vi "main_cn.vi"() -> ()   [LabVIEW 2016]
uses:
  Controls/ExtRefSource.ctl
  Controls/Auto range.ctl
  UI functions/Main_UI_Var.ctl
  <instrlib>/Zurich Instruments LabOne/Public/ziTypeHandle.ctl
  Controls/zi_node.ctl
  UI functions/Main_FUN-Numeric_Var.ctl
  <instrlib>/Zurich Instruments LabOne/Public/Data/ziTypeDemodSampleSingle.ctl
  <instrlib>/Zurich Instruments LabOne/Public/Configure/ziSetValueDouble.vi
  <instrlib>/Zurich Instruments LabOne/Public/Configure/ziSetValueDoubleArray.vi
  <instrlib>/Zurich Instruments LabOne/Zurich Instruments LabOne.lvlib
panel:
  out "Label.Text":string
  in  "FUN-Numeric_Var":T1 {"ZI Handle"."Handle" format="0x%08x"; "ZI Handle"."Conn" format="0x%08x"}
  in  "sigouts/0/imp50":bool caption="50 Ω"
  in  "Address":string="DEV3505"
  in  "stop":bool
  in  "extrefs/0/enable":T4 caption="参考时钟"
  in  "Offset":dbl format="%#_3p"
  in  "Enable":bool
  in  "sigins/0/float":bool caption="Float"
  in  "sigins/0/diff":bool caption="差分"
  in  "sigins/0/imp50":bool caption="50 Ω"
  in  "sigins/0/ac":bool caption="AC"
  in  "sigins/0/autorange":T5=TRUE caption="Boolean"
  in  "sigouts/0/amplitudes/0":dbl=1.0 caption="输出幅值" format="%.2p Vpk"
  in  "sigouts/0/offset":dbl caption="偏置" format="%.2p V"
  in  "sigouts/0/range":dbl(ring)=1.0 caption="输出范围" items=["10 mV"=0.01, "100 mV"=0.1, "1 V"=1.0, "10 V"=10.0]
  in  "sigouts/0/enables/0":bool caption="启用"
  in  "demods/0/rate":dbl=52.31584930419922 caption="数据传输速率" format="%#.3p Sa/s"
  in  "sigouts/0/on":bool caption="启用"
  out "Title_SIG OUT":string
  out "Title_Demodulators":string
  out "Top_Left":bool
  in  "oscs/0/freq":dbl=99999.99999990905 caption="频率" format="%.8p"
  in  "demods/0/timeconstant":dbl(slide)=0.001 caption="时间常数" scale=3e-07..2.0
  in  "demods/0/harmonic":dbl=1.0 caption="谐波" min=1.0 max=1000.0 step=1.0 format="%#_1g"
  in  "demods/0/order":dbl(ring)=4.0 caption="阶次" items=["1"=1.0, "2"=2.0, "3"=3.0, "4"=4.0, "5"=5.0, "6"=6.0, "7"=7.0, "8"=8.0]
  in  "sigins/0/range":dbl=1.0 caption="量程" format="%.1p V"
  in  "参考时钟":u16(ring) items=["Internal Ref", "External Ref/Aux", "External Ref/DIO", "External Ref/Trigger"]
  out "Title_SIG IN":string
  out "Mid_Left":bool
  in  "UI_Var":T6 caption="Var" {"ZI Handle"."Handle" format="0x%08x"; "ZI Handle"."Conn" format="0x%08x"}
  out "X":dbl format="%.5p V"
  out "Mid_Mid":bool caption="Mid_Left"
  out "Y":dbl format="%.5p V"
  out "Mid_Right":bool caption="Mid_Left"
  in  "Preset":u16(ring) items=["Cartesian", "Polar"]
  out "Scope 3":dbl[](graph)
  out "Bottom_Left":bool caption="Mid_Left"
  out "Plotter(R&theta)":waveform(dbl)[](graph) caption="Plotter"
  out "Bottom_Right":bool caption="Mid_Left"
  out "Plotter(XY)":waveform(dbl)[](graph) caption="Plotter"
  # "For development only"
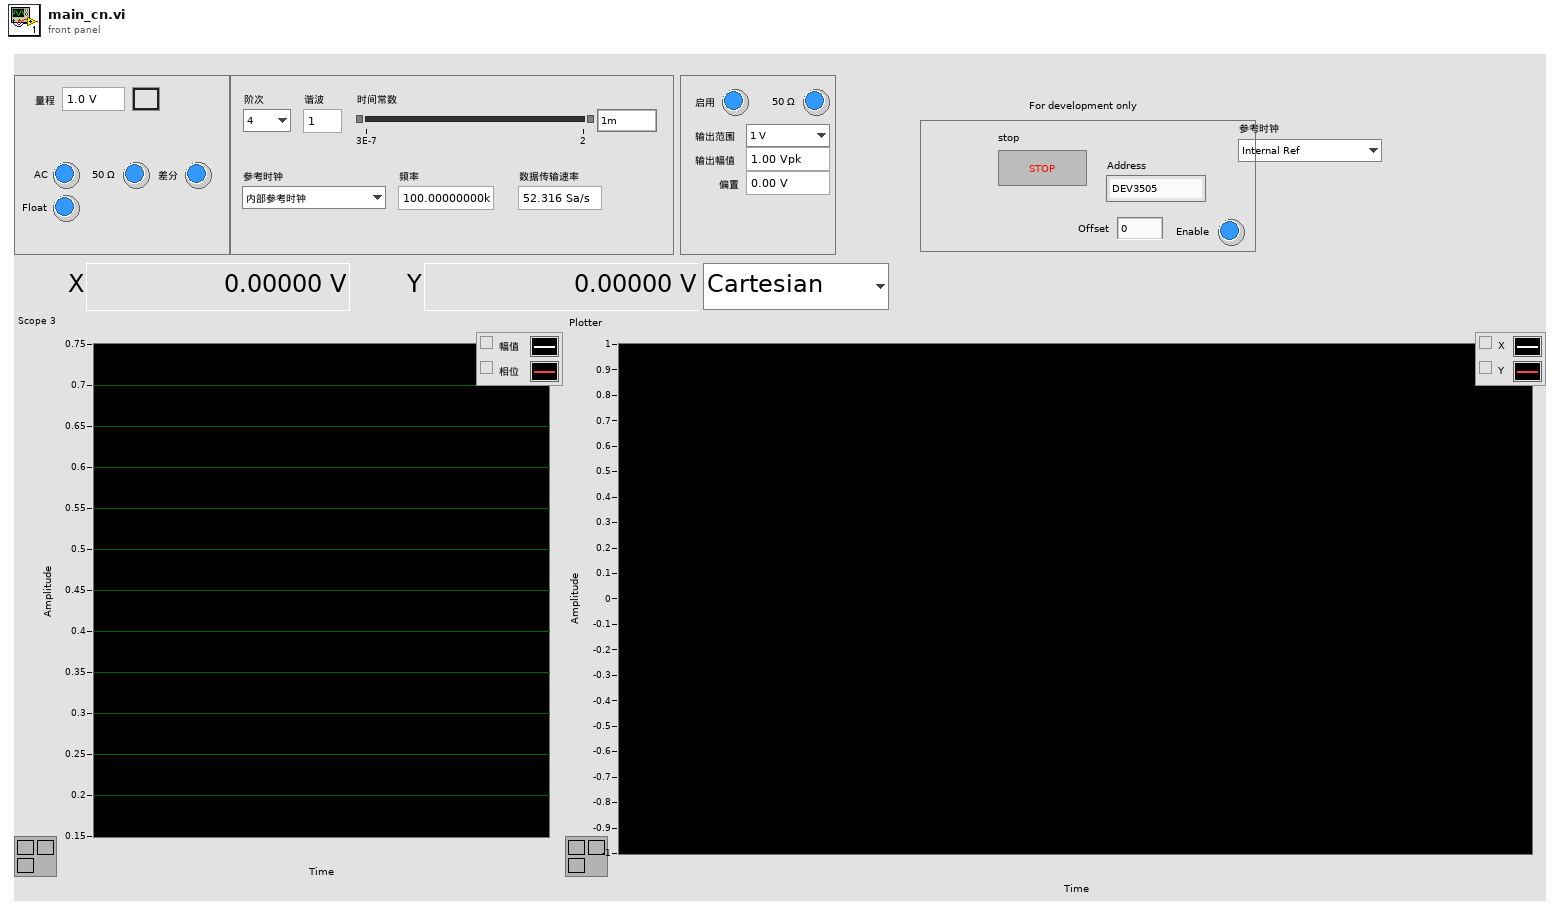
[diagram p1: front panel]
types:
  T1 = typedef "Main_FUN-Numeric_Var.ctl" = cluster{"ZI Handle":T2, "Demod Sample":T3}
  T2 = typedef "Zurich Instruments LabOne.lvlib/ziTypeHandle.ctl" = cluster{"handleValid":bool, "Conn":u64, "Path Prefix":string, "Handle":u64, "Connected":bool, "Clockbase(s)":dbl}
  T3 = typedef "Zurich Instruments LabOne.lvlib/ziTypeDemodSampleSingle.ctl" = cluster{"Timestamps (ticks)":u64, "X (Vrms)":dbl, "Y (Vrms)":dbl, "Osc Phase (deg)":dbl, "Freq (Hz)":dbl, "DIO":u32, "AuxIn0 (V)":dbl, "AuxIn1 (V)":dbl, "Trigger":u32}
  T4 = typedef "ExtRefSource.ctl" = enum16{"内部参考时钟", "外部参考时钟/Aux Input 1", "外部参考时钟/Trigger 1"}
  T5 = typedef "Auto range.ctl" = bool
  T6 = typedef "Main_UI_Var.ctl" = cluster{"ZI Handle":T2, "ZI_node":T7}
  T7 = typedef "zi_node.ctl" = cluster{"Node":string[], "Value":dbl[]}
  T8 = typedef "UI_Queue_Data Type" = cluster{"Cmd":string, "Value":variant}
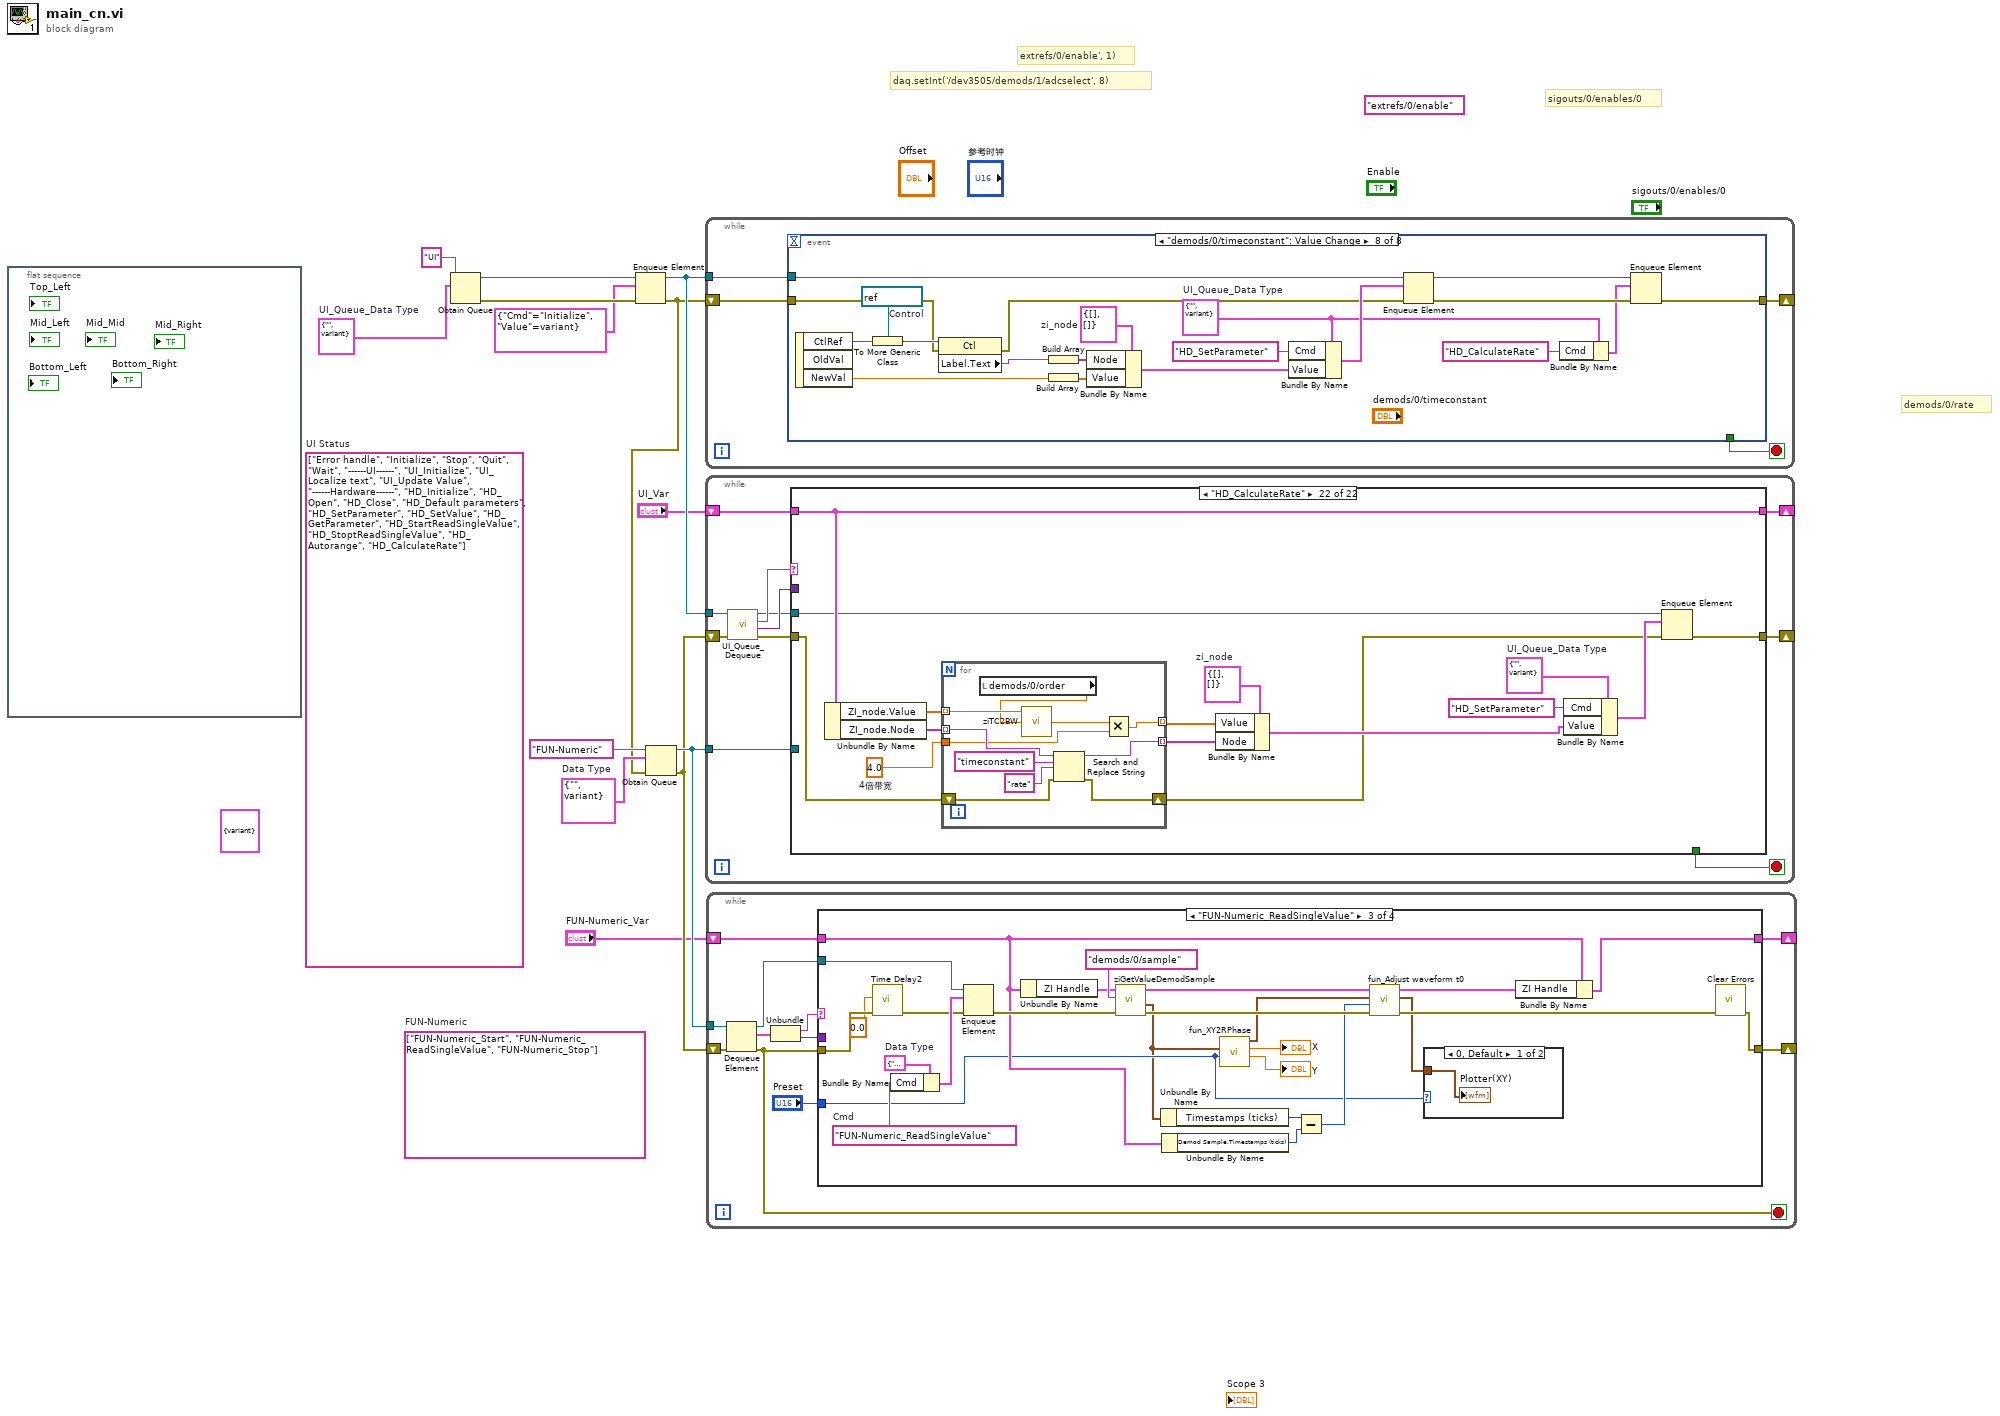
[diagram p0: block diagram]
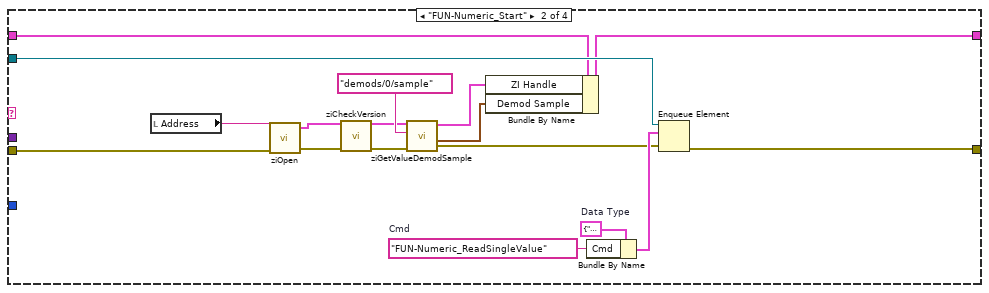
[diagram p3: hidden frame]
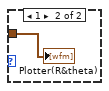
[diagram p4: hidden frame]
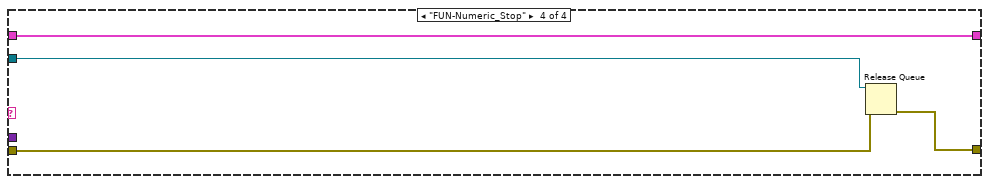
[diagram p5: hidden frame]
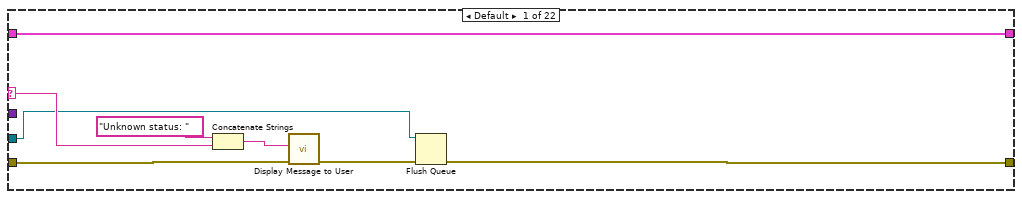
[diagram p6: hidden frame]
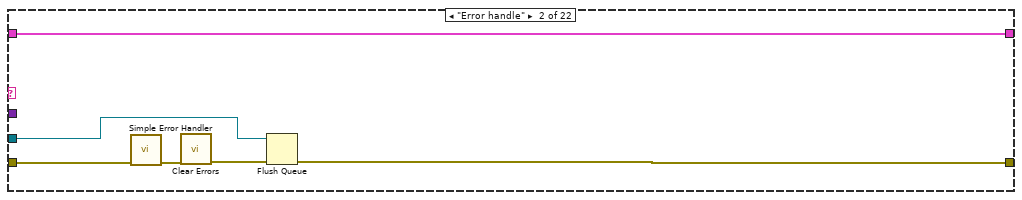
[diagram p7: hidden frame]
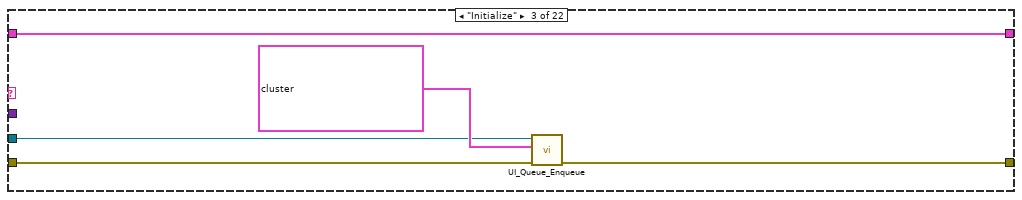
[diagram p8: hidden frame]
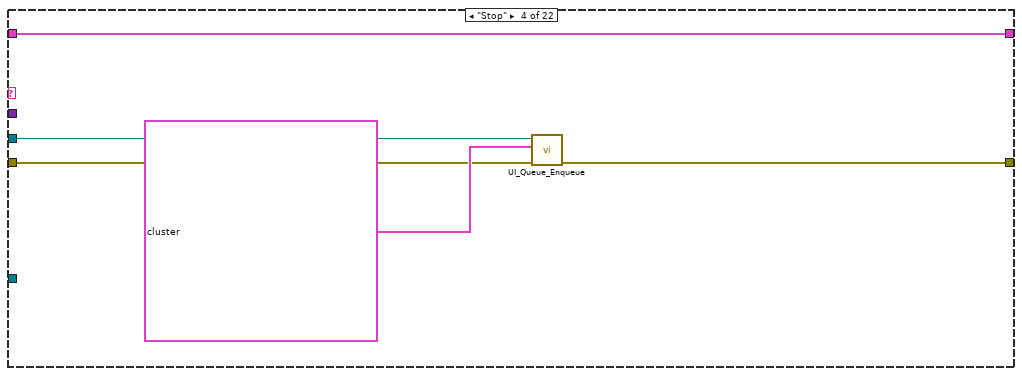
[diagram p9: hidden frame]
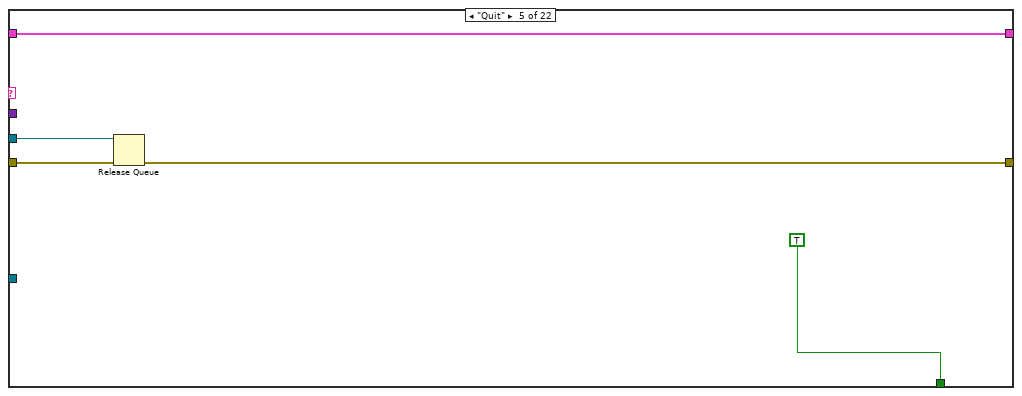
[diagram p10: hidden frame]
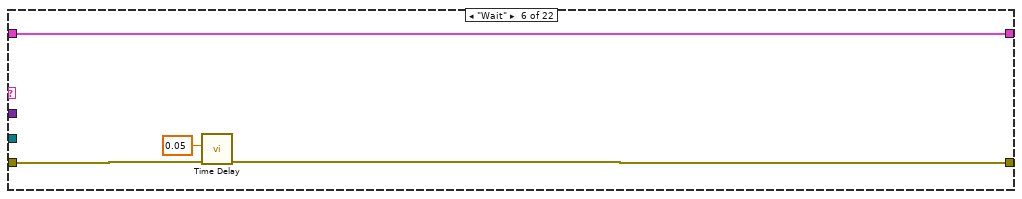
[diagram p11: hidden frame]
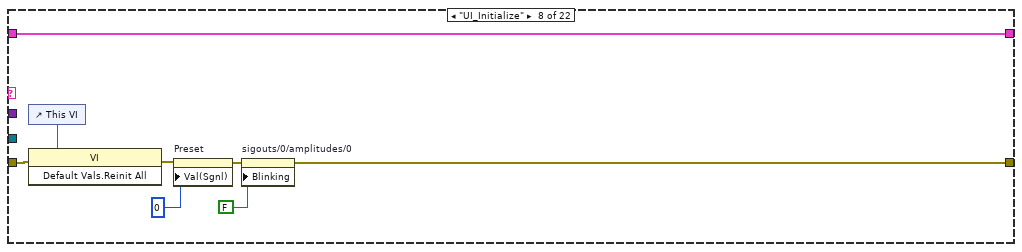
[diagram p13: hidden frame]
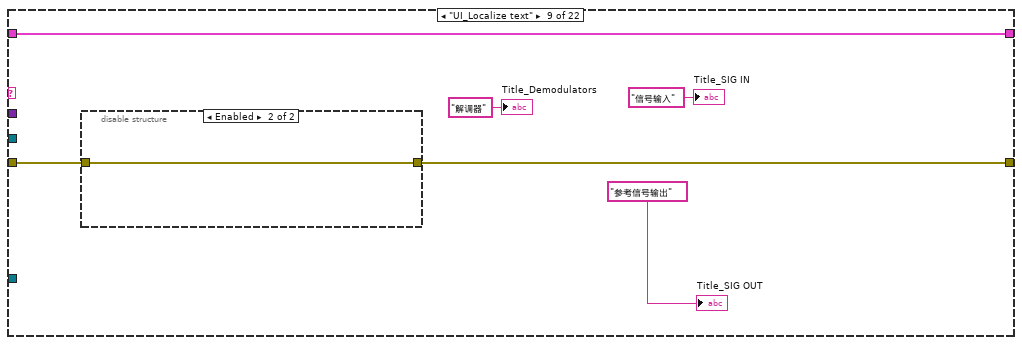
[diagram p14: hidden frame]
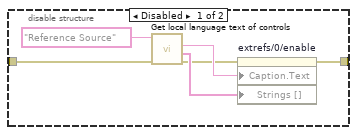
[diagram p15: hidden frame]
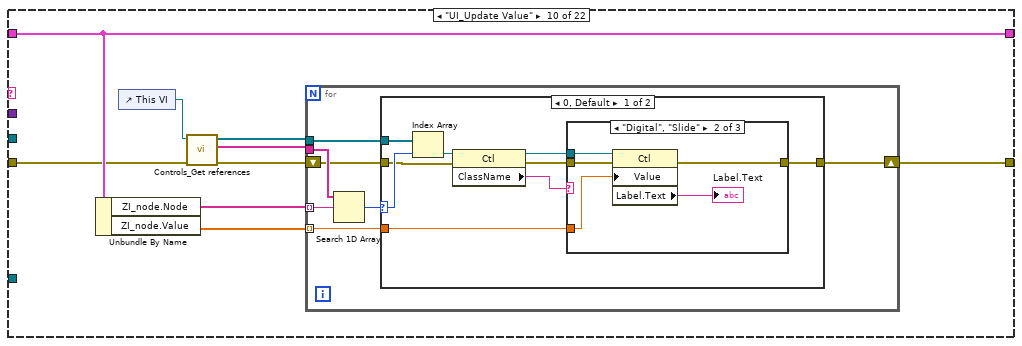
[diagram p16: hidden frame]
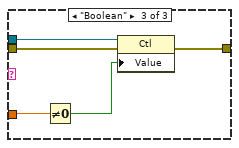
[diagram p18: hidden frame]
diagram:
  (unwired) "extrefs/0/enable"
  w5 = cluster{"Cmd":string, "Value":variant} {"Cmd"="", "Value"=variant}  # Data Type
  (unwired) cluster{"Value":variant} {"Value"=variant} ("element")
  (unwired) string[] ["FUN-Numeric_Start", "FUN-Numeric_ReadSingleValue", "FUN-Numeric_Stop"]  # FUN-Numeric
  (unwired) string[] ["Error handle", "Initialize", "Stop", "Quit", "Wait", "------UI------", "UI_Initialize", "UI_Localize text", "UI_Update Value", "------Hardware------", "HD_Initialize", "HD_Open", "HD_Close", "HD_Default parameters", "HD_SetParameter", "HD_SetValue", "HD_GetParameter", "HD_StartReadSingleValue", "HD_StoptReadSingleValue", "HD_Autorange", "HD_CalculateRate"]  # UI Status
  w6 = T8 {"Cmd"="", "Value"=variant}  # UI_Queue_Data Type
  # "daq.setInt('/dev3505/demods/1/adcselect', 8)"
  # "extrefs/0/enable', 1)"
  # "demods/0/rate"
  # "sigouts/0/enables/0"
  n1 = flat-sequence {
    frame #0 {
    }
  }
  n2 = Obtain Queue(name (unnamed)="UI", element data type=w6) -> (queue out=w12:refnum<queue>, error out=w11:errorcluster)  [unwired: 3 in, 1 out]
  n3 = Enqueue Element(queue=w12, element=cluster{"Cmd":string, "Value":variant} {"Cmd"="Initialize", "Value"=variant}, error in (no error)=w11) -> (queue out=w10:refnum<queue>, error out=w2:errorcluster)  [unwired: 1 in, 1 out]
  n4 = Obtain Queue(name (unnamed)="FUN-Numeric", element data type=w5, error in (no error)=w2) -> (queue out=w4:refnum<queue>, error out=w3:errorcluster)  [unwired: 2 in, 1 out]
  n5 = while {
    tunnel: w10 -> [w17]
    shift-right: [w14] -> _
    shift-left: w2 -> [w15]
    stop <- w16 stop-if-true
    n6 = event shown="[7] \"demods/0/timeconstant\": Value Change" {
      selector: _ -> [_ _ _ _ _ _ _ _]
      dyn-events: _ -> [_ _ _ _ _ _ _ _]
      timeout: _ -> [_ _ _ _ _ _ _ _]
      tunnel: [_ "stop" _ _ _ _ _ _] -> w16
      tunnel: w17 -> [_ w22 _ w59 w76 w91 w102 w122]
      tunnel: w15 -> [w18 w20 _ w43 w64 w78 w95 w111]
      tunnel: [w18 w19 _ w49 w69 _ _ w104] -> w14
      event Timeout {
        n7 = event-data() -> ()  [unwired: 1 in, 3 out]
      }
      event "stop": Value Change {
        n8 = event-data() -> ()  [unwired: 1 in, 6 out]
        n9 = Enqueue Element(queue=w22, element=cluster{"Cmd":string, "Value":variant} {"Cmd"="Stop", "Value"=variant}, error in (no error)=w20) -> (error out=w19:errorcluster)  [unwired: 1 in, 2 out]
      }
      event "Preset": Value Change {
        n10 = event-data() -> ("NewVal"=w26:u16)  [unwired: 1 in]
        n11 = invoke on="Plotter(XY)" class="WFChart (strict)" method="Reinit To Default"() -> ()  [unwired: 3 in, 3 out]
        n12 = case shown="0, Default" w26 {
          tunnel: ["%.5p V" "%.5p V"] -> w30
          tunnel: ["%.5p deg" "%.5p V"] -> w29
          tunnel: ["幅值" "X"] -> w28
          tunnel: ["相位" "Y"] -> w27
          frame 1 {
          }
          frame 0, Default {
          }
        }
        n13 = property on="X" class="DigNum (strict)"("Caption.Text"=w28) -> ()  [unwired: 2 in, 2 out]
        n14 = property on="Y" class="DigNum (strict)"("Caption.Text"=w27) -> ()  [unwired: 2 in, 2 out]
        n15 = property on="X" class="DigNum (strict)"("FormatString"=w30) -> ()  [unwired: 2 in, 2 out]
        n16 = property on="Y" class="DigNum (strict)"("FormatString"=w29) -> ()  [unwired: 2 in, 2 out]
        n17 = case shown="1" w26 {
          tunnel: [TRUE FALSE] -> w25
          tunnel: [FALSE TRUE] -> w24
          frame 0, Default {
          }
          frame 1 {
          }
        }
        n18 = property on="Plotter(XY)" class="WFChart (strict)"("Visible"=w25) -> ()  [unwired: 2 in, 2 out]
        n19 = property on="Plotter(R&theta)" class="WFChart (strict)"("Visible"=w24) -> ()  [unwired: 2 in, 2 out]
      }
      event "sigouts/0/on", "sigins/0/diff", "sigins/0/imp50", "sigins/0/ac", "sigouts/0/imp50", "sigins/0/float": Value Change {
        w47 = refnum<vi> refnum  # Control
        w53 = T8 {"Cmd"="", "Value"=variant}  # UI_Queue_Data Type
        w58 = T7 {"Node"=[], "Value"=[]}  # zi_node
        n20 = event-data() -> ("CtlRef"=w46:refnum<vi>, "NewVal"=w56:bool)  [unwired: 1 in, 4 out]
        n21 = To More Generic Class(target class=w47, reference=w46) -> (generic class reference=w48:refnum<vi>)
        n22 = property class="Ctl"(reference=w48, error in=w43) -> (error out=w44:errorcluster, "Label.Text"=w45:string)  [unwired: 1 out]
        n23 = Boolean To (0,1)(Boolean=w56) -> (0, 1=w54:i16)
        n24 = Build Array(w45) -> (w57:string[])
        n25 = Build Array(w54) -> (w55:i16[])
        n26 = Bundle By Name(cluster=w58, "Node"=w57, "Value"=w55) -> (w51:T7)
        n27 = Bundle By Name(cluster=w53, "Cmd"="HD_SetParameter", "Value"=w51) -> (w52:T8)
        n28 = Enqueue Element(queue=w59, element=w52, error in (no error)=w44) -> (error out=w49:errorcluster)  [unwired: 1 in, 2 out]
      }
      event Value Change {
        w67 = refnum<vi> refnum  # Control
        w73 = T8 {"Cmd"="", "Value"=variant}  # UI_Queue_Data Type
        w75 = T7 {"Node"=[], "Value"=[]}  # zi_node
        # "sigins/0/autorange"
        n29 = event-data() -> ("CtlRef"=w66:refnum<vi>)  [unwired: 1 in, 3 out]
        n30 = To More Generic Class(target class=w67, reference=w66) -> (generic class reference=w68:refnum<vi>)
        n31 = property class="Ctl"(reference=w68, error in=w64) -> (error out=w65:errorcluster, "Label.Text"=w61:string)  [unwired: 1 out]
        n32 = Match Pattern(string=w61, regular expression="sigins/[0-9]") -> (match substring=w60:string)  [unwired: 1 in, 3 out]
        n33 = Build Array(w60) -> (w74:string[])
        n34 = Bundle By Name(cluster=w75, "Node"=w74, "Value"=dbl[] [1.0]) -> (w71:T7)
        n35 = Bundle By Name(cluster=w73, "Cmd"="HD_Autorange", "Value"=w71) -> (w72:T8)
        n36 = Enqueue Element(queue=w76, element=w72, error in (no error)=w65) -> (error out=w69:errorcluster)  [unwired: 1 in, 2 out]
      }
      event "sigouts/0/amplitudes/0", "demods/0/rate", "oscs/0/freq", "demods/0/order", "demods/0/harmonic", "sigins/0/range", "sigouts/0/range", "sigouts/0/offset": Value Change {
        w80 = refnum<vi> refnum  # Control
        w88 = T8 {"Cmd"="", "Value"=variant}  # UI_Queue_Data Type
        w90 = T7 {"Node"=[], "Value"=[]}  # zi_node
        n37 = event-data() -> ("CtlRef"=w82:refnum<vi>, "NewVal"=w84:dbl)  [unwired: 1 in, 4 out]
        n38 = To More Generic Class(target class=w80, reference=w82) -> (generic class reference=w81:refnum<vi>)
        n39 = property class="Ctl"(reference=w81, error in=w78) -> (error out=w77:errorcluster, "Label.Text"=w79:string)  [unwired: 1 out]
        n40 = Build Array(w79) -> (w89:string[])
        n41 = Build Array(w84) -> (w83:dbl[])
        n42 = Bundle By Name(cluster=w90, "Node"=w89, "Value"=w83) -> (w86:T7)
        n43 = Bundle By Name(cluster=w88, "Cmd"="HD_SetParameter", "Value"=w86) -> (w87:T8)
        n44 = Enqueue Element(queue=w91, element=w87, error in (no error)=w77) -> ()  [unwired: 1 in, 3 out]
      }
      event Value Change {
        w96 = refnum<vi> refnum  # Control
        w101 = T8 {"Cmd"="", "Value"=variant}  # UI_Queue_Data Type
        n45 = event-data() -> ("CtlRef"=w98:refnum<vi>, "NewVal"=w93:T4)  [unwired: 1 in, 4 out]
        n46 = To More Generic Class(target class=w96, reference=w98) -> (generic class reference=w97:refnum<vi>)
        n47 = property class="Ctl" props=["Label", "Text"](reference=w97, error in=w95) -> (error out=w94:errorcluster)  [unwired: 2 out]
        n48 = call "ExtRefSource_set.vi"("extrefs/0/enable"=w93) -> ("zi_node"=w92:T7)  [unwired: 10 in]
        n49 = Bundle By Name(cluster=w101, "Cmd"="HD_SetParameter", "Value"=w92) -> (w100:T8)
        n50 = Enqueue Element(queue=w102, element=w100, error in (no error)=w94) -> ()  [unwired: 1 in, 3 out]
      }
      event "demods/0/timeconstant": Value Change {
        w112 = refnum<vi> refnum  # Control
        w107 = T8 {"Cmd"="", "Value"=variant}  # UI_Queue_Data Type
        w121 = T7 {"Node"=[], "Value"=[]}  # zi_node
        n51 = event-data() -> ("CtlRef"=w114:refnum<vi>, "NewVal"=w116:dbl)  [unwired: 1 in, 1 out]
        n52 = To More Generic Class(target class=w112, reference=w114) -> (generic class reference=w113:refnum<vi>)
        n53 = property class="Ctl"(reference=w113, error in=w111) -> (error out=w110:errorcluster, "Label.Text"=w109:string)  [unwired: 1 out]
        n54 = Build Array(w109) -> (w120:string[])
        n55 = Build Array(w116) -> (w115:dbl[])
        n56 = Bundle By Name(cluster=w121, "Node"=w120, "Value"=w115) -> (w118:T7)
        n57 = Bundle By Name(cluster=w107, "Cmd"="HD_SetParameter", "Value"=w118) -> (w119:T8)
        n58 = Enqueue Element(queue=w122, element=w119, error in (no error)=w110) -> (queue out=w106:refnum<queue>, error out=w105:errorcluster)  [unwired: 1 in, 1 out]
        n59 = Bundle By Name(cluster=w107, "Cmd"="HD_CalculateRate") -> (w103:T8)
        n60 = Enqueue Element(queue=w106, element=w103, error in (no error)=w105) -> (error out=w104:errorcluster)  [unwired: 1 in, 2 out]
      }
    }
  }
  n61 = while {
    tunnel: w10 -> [w133]
    shift-right: [w127] -> _
    shift-left: w3 -> [w132]
    shift-right: [w124] -> _
    shift-left: "UI_Var" -> [w125]
    tunnel: w4 -> [w123]
    stop <- w126 stop-if-true
    n62 = call "UI_Queue_Dequeue.vi"("error in (no error)"=w132, "UI Queue in"=w133) -> ("error out"=w130:errorcluster, "Value"=w129:variant, "Cmd"=w131:string, "UI Queue out"=w128:refnum<queue>)  [unwired: 6 in]
    n63 = case shown="\"HD_CalculateRate\"" w131 {
      selector: w131 -> [w140 _ _ _ _ _ _ _ _ _ _ _ _ _ _ _ _ _ _ _ _ _]
      tunnel: w130 -> [w141 w147 w151 w156 w162 w165 w168 w172 w179 w190 w228 w232 w240 w246 w257 w270 w286 w299 w308 w316 w336 w349]
      tunnel: w129 -> [_ _ _ _ _ _ _ _ _ _ _ _ _ _ _ _ w293 _ _ _ w335 _]
      tunnel: w128 -> [w138 w143 w149 w154 w161 _ _ _ _ _ _ w229 _ _ w250 w272 w288 _ _ _ w325 w356]
      tunnel: [w139 w144 w150 w155 w160 w164 w168 w170 w178 w192 w228 w231 w236 w245 w252 w273 w290 w300 w311 w315 w323 w355] -> w127
      tunnel: [_ _ _ _ TRUE _ _ _ _ _ _ _ _ _ _ _ _ _ _ _ _ _] -> w126
      tunnel: w125 -> [w137 w142 w148 w153 w158 w166 w167 w176 w177 w191 w227 w233 w239 w243 w260 w271 w289 w306 w312 w320 w334 w359]
      tunnel: [w137 w142 w148 w153 w158 w166 w167 w176 w177 w191 w227 w233 w238 w247 w261 w269 w285 w304 w312 w320 w330 w359] -> w124
      tunnel: w123 -> [_ _ _ _ _ _ _ _ _ _ _ _ _ _ _ _ _ _ w309 w314 _ _]
      frame Default {
        n64 = Concatenate Strings("Unknown status: " ("string"), w140) -> (w136:string)
        n65 = call "Display Message to User"("error in (no error)"=w141, "Message"=w136) -> ("error out"=w134:errorcluster)  [unwired: 8 in, 1 out]
        n66 = Flush Queue(queue=w138, error in (no error)=w134) -> (error out=w139:errorcluster)  [unwired: 2 out]
      }
      frame "Error handle" {
        n67 = call <vilib>:"Simple Error Handler.vi"("error in (no error)"=w147) -> ("error out"=w146:errorcluster)  [unwired: 4 in, 4 out]
        n68 = call <vilib>:"Clear Errors.vi"("error in (no error)"=w146) -> ("error out"=w145:errorcluster)  [unwired: 5 in, 1 out]
        n69 = Flush Queue(queue=w143, error in (no error)=w145) -> (error out=w144:errorcluster)  [unwired: 2 out]
      }
      frame "Initialize" {
        n70 = call "UI_Queue_Enqueue.vi"("error in (no error)"=w151, "UI Commands"=cluster{"Cmd":string, "Value":variant}[] [{"Cmd"="UI_Initialize", "Value"=variant}, {"Cmd"="UI_Localize text", "Value"=variant}, {"Cmd"="HD_Initialize", "Value"=variant}], "Queue in"=w149) -> ("error out"=w150:errorcluster)  [unwired: 7 in, 1 out]
      }
      frame "Stop" {
        n71 = call "UI_Queue_Enqueue.vi"("error in (no error)"=w156, "UI Commands"=cluster{"Cmd":string, "Value":variant}[] [{"Cmd"="HD_StoptReadSingleValue", "Value"=variant}, {"Cmd"="HD_Close", "Value"=variant}, {"Cmd"="Quit", "Value"=variant}], "Queue in"=w154) -> ("error out"=w155:errorcluster)  [unwired: 7 in, 1 out]
      }
      frame "Quit" {
        n72 = Release Queue(queue=w161, error in (no error)=w162) -> (error out=w160:errorcluster)  [unwired: 1 in, 2 out]
      }
      frame "Wait" {
        n73 = call "Time Delay"("error in (no error)"=w165, "Delay Time (s)"=0.05) -> ("error out"=w164:errorcluster)  [unwired: 9 in]
      }
      frame "------UI------" {
      }
      frame "UI_Initialize" {
        n74 = control-ref of="This VI"() -> (w174:refnum<vi>)
        n75 = invoke class="VI" method="Default Vals.Reinit All"(reference=w174, error in=w172) -> (error out=w173:errorcluster)  [unwired: 1 in, 2 out]
        n76 = property on="Preset" class="Ring (strict)"(error in=w173, "Val(Sgnl)"=u16 0 ("Value (Signaling)")) -> (error out=w171:errorcluster)  [unwired: 1 in, 1 out]
        n77 = property on="sigouts/0/amplitudes/0" class="DigNum (strict)"(error in=w171, "Blinking"=FALSE) -> (error out=w170:errorcluster)  [unwired: 1 in, 1 out]
      }
      frame "UI_Localize text" {
        n78 = disable-structure shown="Enabled" {
          disable-tunnel: w179 -> [w184 w189]
          disable-tunnel: [w183 w189] -> w178
          frame Disabled {
            n79 = call "Get local language text of controls.vi"("error in (no error)"=w184, "Control Label"="Reference Source") -> ("error out"=w185:errorcluster, "Values"=w187:string[], "Control Caption"=w186:string)  [unwired: 6 in, 1 out]
            n80 = property on="extrefs/0/enable" class="Enum (strict)"(error in=w185, "Caption.Text"=w186, "Strings []"=w187) -> (error out=w183:errorcluster)  [unwired: 1 in, 1 out]
          }
          frame Enabled {
          }
        }
        "Title_SIG IN" <- "信号输入" ("Title_SIG IN")
        "Title_Demodulators" <- "解调器" ("Title_SIG IN 2")
        "Title_SIG OUT" <- "参考信号输出" ("Title_SIG OUT")
      }
      frame "UI_Update Value" {
        n81 = Unbundle By Name(w191) -> ("ZI_node.Node"=w197:string[], "ZI_node.Value"=w193:dbl[])
        n82 = control-ref of="This VI"() -> (w198:refnum<vi>)
        n83 = call "Controls_Get references.vi"("error in (no error)"=w190, "VI in"=w198) -> ("error out"=w194:errorcluster, "Labels of Controls"=w196:string[], "References of Controls"=w195:refnum<vi>[])  [unwired: 7 in]
        n84 = for {
          tunnel: w197 -> [w204] mode=indexing
          tunnel: w196 -> [w205]
          tunnel: w195 -> [w202]
          tunnel: w193 -> [w200] mode=indexing
          shift-right: [w199] -> w192
          shift-left: w194 -> [w201]
          n85 = Search 1D Array(1D array=w205, element=w204) -> (index of element=w203:i32)  [unwired: 1 in]
          n86 = case shown="0, Default" w203 {
            selector: w203 -> [w214 _]
            tunnel: w202 -> [w213 _]
            tunnel: w201 -> [w212 w226]
            tunnel: w200 -> [w206 _]
            tunnel: [w209 w226] -> w199
            frame 0, Default {
              n87 = Index Array(array=w213, index=w214) -> (element=w211:refnum<vi>)
              n88 = property class="Ctl"(reference=w211, error in=w212) -> (reference out=w208:refnum<vi>, error out=w210:errorcluster, "ClassName"=w207:string)
              n89 = case shown="\"Digital\", \"Slide\"" w207 {
                tunnel: w210 -> [w215 w220 w225]
                tunnel: [w215 w219 w224] -> w209
                tunnel: w208 -> [_ w218 w223]
                tunnel: w206 -> [_ w217 w222]
                frame Default {
                }
                frame "Digital", "Slide" {
                  n90 = property class="Ctl"(reference=w218, error in=w220, "Value"=w217) -> (error out=w219:errorcluster, "Label.Text"=→"Label.Text":string)  [unwired: 1 out]
                }
                frame "Boolean" {
                  n91 = Not Equal To 0?(x=w222) -> (x != 0?=w221:bool)
                  n92 = property class="Ctl"(reference=w223, error in=w225, "Value"=w221) -> (error out=w224:errorcluster)  [unwired: 1 out]
                }
              }
            }
            frame -1 {
            }
          }
        }
      }
      frame "------Hardware------" {
      }
      frame "HD_Initialize" {
        # "HD_StartReadSingleValue"
        n93 = call "UI_Queue_Enqueue.vi"("error in (no error)"=w232, "UI Commands"=cluster{"Cmd":string, "Value":variant}[] [{"Cmd"="HD_Open", "Value"=variant}, {"Cmd"="HD_Default parameters", "Value"=variant}, {"Cmd"="HD_StartReadSingleValue", "Value"=variant}], "Queue in"=w229) -> ("error out"=w231:errorcluster)  [unwired: 7 in, 1 out]
      }
      frame "HD_Open" {
        n94 = call <instrlib>:"ziOpen.vi"("Error In"=w240, "Address"="Address") -> ("Error Out"=w237:errorcluster, "HandleOut"=w235:T2)  [unwired: 2 in, 1 out]
        n95 = call <instrlib>:"ziCheckVersion.vi"("Handle In"=w235, "Error In"=w237) -> ("Handle Out"=w234:T2, "Error Out"=w236:errorcluster)  [unwired: 11 in, 1 out]
        n96 = Bundle By Name(cluster=w239, "ZI Handle"=w234) -> (w238:T6)
      }
      frame "HD_Close" {
        n97 = Unbundle By Name(w243) -> ("ZI Handle"=w242:T2)
        n98 = call <instrlib>:"ziClose.vi"("Error In"=w246, "Handle In"=w242) -> ("Error Out"=w245:errorcluster, "Handle Out"=w244:T2)  [unwired: 2 in]
        n99 = Bundle By Name(cluster=w243, "ZI Handle"=w244) -> (w247:T6)
      }
      frame "HD_Default parameters" {
        n100 = Unbundle By Name(w260) -> ("ZI Handle"=w258:T2)
        n101 = call-poly <instrlib>:"ziSetValue.vi"("Error In"=w257, "Value"=0.0, "Path"="sigouts/0/on", "Handle In"=w258) -> ("Error Out"=w256:errorcluster, "Handle Out"=w248:T2)  [unwired: 1 in]
        n102 = call "Lock-in Default parameters.vi"("error in (no error)"=w256, "Handle in"=w248) -> ("error out"=w251:errorcluster, "zi_node"=w249:T7, "Handle out"=w259:T2)  [unwired: 7 in]
        n103 = Bundle By Name(cluster=w260, "ZI Handle"=w259, "ZI_node"=w249) -> (w261:T6)
        n104 = for {
          tunnel: cluster{"Cmd":string, "Value":variant}[] [{"Cmd"="HD_GetParameter", "Value"=variant}, {"Cmd"="Wait", "Value"=variant}] ("UI Commands") -> [w265] mode=indexing
          tunnel: w250 -> [w262]
          shift-right: [w264] -> w252
          shift-left: w251 -> [w263]
          n105 = Enqueue Element At Opposite End(queue=w262, element=w265, error in (no error)=w263) -> (error out=w264:errorcluster)  [unwired: 1 in, 2 out]
        }
      }
      frame "HD_GetParameter" {
        n106 = Unbundle By Name(w271) -> ("ZI_node.Node"=w267:string[])
        n107 = for {
          tunnel: w267 -> [w280] mode=indexing
          shift-right: [w282] -> w274
          shift-left: w270 -> [w283]
          tunnel: [w279] -> w266 mode=indexing
          shift-right: [w277] -> w275
          shift-left: w271 -> [w278]
          n108 = Unbundle By Name(w278) -> ("ZI Handle"=w281:T2)
          n109 = call <instrlib>:"ziGetValueDouble.vi"("error in"=w283, "Path"=w280, "Handle in"=w281) -> ("error out"=w282:errorcluster, "Value"=w279:dbl, "Handle out"=w276:T2)
          n110 = Bundle By Name(cluster=w278, "ZI Handle"=w276) -> (w277:T6)
        }
        n111 = Bundle By Name(cluster=w275, "ZI_node.Node"=w267, "ZI_node.Value"=w266) -> (w269:T6)
        n112 = Enqueue Element(queue=w272, element=cluster{"Cmd":string, "Value":variant} {"Cmd"="UI_Update Value", "Value"=variant}, error in (no error)=w274) -> (error out=w273:errorcluster)  [unwired: 1 in, 2 out]
      }
      frame "HD_SetParameter" {
        w292 = T7 {"Node"=[], "Value"=[]}  # zi_node
        n113 = Variant To Data(error in=w286, type=w292, Variant=w293) -> (data=w284:T7, error out=w287:errorcluster)
        n114 = Bundle By Name(cluster=w289, "ZI_node"=w284) -> (w285:T6)
        n115 = for {
          tunnel: cluster{"Cmd":string, "Value":variant}[] [{"Cmd"="HD_SetValue", "Value"=variant}, {"Cmd"="Wait", "Value"=variant}, {"Cmd"="HD_GetParameter", "Value"=variant}] ("UI Commands") -> [w295] mode=indexing
          shift-right: [w297] -> w290
          shift-left: w287 -> [w296]
          tunnel: w288 -> [w294]
          n116 = Enqueue Element(queue=w294, element=w295, error in (no error)=w296) -> (error out=w297:errorcluster)  [unwired: 1 in, 2 out]
        }
      }
      frame "HD_SetValue" {
        # "Can be replaced by \"Double Array\""
        n117 = Unbundle By Name(w306) -> ("ZI Handle"=w305:T2, "ZI_node"=w298:T7)
        n118 = Unbundle By Name(w298) -> ("Node"=w302:string[], "Value"=w303:dbl[])
        n119 = call-poly <instrlib>:"ziSetValue.vi"("Error In"=w299, "Values"=w303, "Paths"=w302, "Handle In"=w305) -> ("Error Out"=w300:errorcluster, "Handle Out"=w301:T2)  [unwired: 1 in]
        n120 = Bundle By Name(cluster=w306, "ZI Handle"=w301, "ZI_node"=w298) -> (w304:T6)
      }
      frame "HD_StartReadSingleValue" {
        w310 = cluster{"Cmd":string, "Value":variant} {"Cmd"="", "Value"=variant}  # Data Type
        w313 = "FUN-Numeric_Start"  # Cmd
        n121 = Bundle By Name(cluster=w310, "Cmd"=w313) -> (w307:cluster{"Cmd":string, "Value":variant})
        n122 = Enqueue Element(queue=w309, element=w307, error in (no error)=w308) -> (error out=w311:errorcluster)  [unwired: 1 in, 2 out]
      }
      frame "HD_StoptReadSingleValue" {
        w318 = cluster{"Cmd":string, "Value":variant} {"Cmd"="", "Value"=variant}  # Data Type
        w317 = "FUN-Numeric_Stop"  # Cmd
        n123 = Bundle By Name(cluster=w318, "Cmd"=w317) -> (w319:cluster{"Cmd":string, "Value":variant})
        n124 = Enqueue Element(queue=w314, element=w319, error in (no error)=w316) -> (error out=w315:errorcluster)  [unwired: 1 in, 2 out]
      }
      frame "HD_Autorange" {
        w327 = string[] ["sigins/0/range"]  # Read changed range
        w337 = T7 {"Node"=[], "Value"=[]}  # zi_node
        n125 = Variant To Data(error in=w336, type=w337, Variant=w335) -> (data=w333:T7, error out=w332:errorcluster)
        n126 = Unbundle By Name(w333) -> ("Node"=w328:string[])
        n127 = Unbundle By Name(w334) -> ("ZI Handle"=w331:T2)
        n128 = for {
          shift-right: [w345] -> w324
          shift-left: w332 -> [w346]
          shift-right: [w343] -> w329
          shift-left: w331 -> [w344]
          tunnel: w328 -> [w342] mode=indexing
          n129 = call <instrlib>:"ziAutoRange.vi"("Error in"=w346, "Path"=w342, "Handle in"=w344) -> ("Error out"=w345:errorcluster, "Handle out"=w343:T2)  [unwired: 6 in, 1 out]
        }
        n130 = call "Time Delay3"("error in (no error)"=w324, "Delay Time (s)"=0.5) -> ("error out"=w322:errorcluster)  [unwired: 9 in]
        n131 = Bundle By Name(cluster=w334, "ZI_node.Node"=w327, "ZI Handle"=w329) -> (w330:T6)
        n132 = for {
          tunnel: cluster{"Cmd":string, "Value":variant}[] [{"Cmd"="HD_GetParameter", "Value"=variant}, {"Cmd"="Wait", "Value"=variant}] ("UI Commands") -> [w339] mode=indexing
          shift-right: [w341] -> w323
          shift-left: w322 -> [w340]
          tunnel: w325 -> [w338]
          n133 = Enqueue Element(queue=w338, element=w339, error in (no error)=w340) -> (error out=w341:errorcluster)  [unwired: 1 in, 2 out]
        }
      }
      frame "HD_CalculateRate" {
        w347 = 4.0  # 4倍带宽
        w353 = T8 {"Cmd"="", "Value"=variant}  # UI_Queue_Data Type
        w354 = T7 {"Node"=[], "Value"=[]}  # zi_node
        n134 = Unbundle By Name(w359) -> ("ZI_node.Value"=w360:dbl[], "ZI_node.Node"=w361:string[])
        n135 = for {
          tunnel: w361 -> [w370] mode=indexing
          shift-right: [w368] -> w348
          shift-left: w349 -> [w369]
          tunnel: w360 -> [w367] mode=indexing
          tunnel: [w363] -> w358 mode=indexing
          tunnel: [w364] -> w357 mode=indexing
          tunnel: w347 -> [w362]
          n136 = local read "demods/0/order"() -> (w366:dbl)
          n137 = call <instrlib>:"ziTC2BW.vi"("Order (1)"=w366, "TC (s)"=w367) -> ("BW (Hz)"=w365:dbl)  [unwired: 1 in]
          n138 = Search and Replace String(input string=w370, search string="timeconstant", replace string="rate" ("replace string (\"\")"), error in=w369) -> (result string=w364:string, error out=w368:errorcluster)  [unwired: 4 in, 2 out]
          n139 = Multiply(x=w365, y=w362) -> (x*y=w363:dbl)
        }
        n140 = Bundle By Name(cluster=w354, "Value"=w358, "Node"=w357) -> (w351:T7)
        n141 = Bundle By Name(cluster=w353, "Cmd"="HD_SetParameter", "Value"=w351) -> (w350:T8)
        n142 = Enqueue Element(queue=w356, element=w350, error in (no error)=w348) -> (error out=w355:errorcluster)  [unwired: 1 in, 2 out]
      }
    }
  }
  n143 = while {
    tunnel: w4 -> [w383]
    shift-right: [w377] -> _
    shift-left: w3 -> [w379]
    shift-right: [w373] -> _
    shift-left: "FUN-Numeric_Var" -> [w374]
    stop <- w378 stop-if-true
    n144 = Dequeue Element(queue=w383, error in (no error)=w379) -> (queue out=w376:refnum<queue>, element=w382:cluster{"Cmd":string, "Value":variant}, error out=w378:errorcluster)  [unwired: 1 in, 1 out]
    n145 = Unbundle(w382) -> ("Cmd"=w381:string, "Value"=w380:variant)
    n146 = case shown="\"FUN-Numeric_ReadSingleValue\"" w381 {
      tunnel: w380 -> [_ _ _ _]
      tunnel: w378 -> [w385 w402 w428 w433]
      tunnel: [w385 w396 w426 w434] -> w377
      tunnel: w376 -> [_ w395 w420 w432]
      tunnel: "Preset" -> [_ _ w405 _]
      tunnel: w374 -> [w384 w390 w415 w431]
      tunnel: [w384 w389 w417 w431] -> w373
      frame "idle", Default {
      }
      frame "FUN-Numeric_Start" {
        w399 = cluster{"Cmd":string, "Value":variant} {"Cmd"="", "Value"=variant}  # Data Type
        w398 = "FUN-Numeric_ReadSingleValue"  # Cmd
        n147 = local read "Address"() -> (w401:string)
        n148 = call <instrlib>:"ziOpen.vi"("Error In"=w402, "Address"=w401) -> ("Error Out"=w394:errorcluster, "HandleOut"=w400:T2)  [unwired: 2 in, 1 out]
        n149 = call <instrlib>:"ziCheckVersion.vi"("Handle In"=w400, "Error In"=w394) -> ("Handle Out"=w391:T2, "Error Out"=w393:errorcluster)  [unwired: 11 in, 1 out]
        n150 = call <instrlib>:"ziGetValueDemodSample.vi"("error in"=w393, "Path"="demods/0/sample", "Handle In"=w391) -> ("error out"=w387:errorcluster, "Demod Sample Out"=w386:T3, "Handle Out"=w388:T2)  [unwired: 2 in]
        n151 = Bundle By Name(cluster=w390, "ZI Handle"=w388, "Demod Sample"=w386) -> (w389:T1)
        n152 = Bundle By Name(cluster=w399, "Cmd"=w398) -> (w397:cluster{"Cmd":string, "Value":variant})
        n153 = Enqueue Element(queue=w395, element=w397, error in (no error)=w387) -> (error out=w396:errorcluster)  [unwired: 1 in, 2 out]
      }
      frame "FUN-Numeric_ReadSingleValue" {
        w425 = cluster{"Cmd":string, "Value":variant} {"Cmd"="", "Value"=variant}  # Data Type
        w424 = "FUN-Numeric_ReadSingleValue"  # Cmd
        n154 = call "Time Delay2"("error in (no error)"=w428, "Delay Time (s)"=0.0) -> ("error out"=w419:errorcluster)  [unwired: 9 in]
        n155 = Bundle By Name(cluster=w425, "Cmd"=w424) -> (w423:cluster{"Cmd":string, "Value":variant})
        n156 = Enqueue Element(queue=w420, element=w423, error in (no error)=w419) -> (error out=w421:errorcluster)  [unwired: 1 in, 2 out]
        n157 = Unbundle By Name(w415) -> ("ZI Handle"=w418:T2)
        n158 = call <instrlib>:"ziGetValueDemodSample.vi"("error in"=w421, "Path"="demods/0/sample", "Handle In"=w418) -> ("error out"=w411:errorcluster, "Demod Sample Out"=w403:T3, "Handle Out"=w410:T2)  [unwired: 2 in]
        n159 = Unbundle By Name(w403) -> ("Timestamps (ticks)"=w414:u64)
        n160 = Unbundle By Name(w415) -> ("Demod Sample.Timestamps (ticks)"=w413:u64)
        n161 = call "fun_XY2RPhase.vi"("Preset"=w405, "Demod Sample Out"=w403) -> ("Y or Phase"=→"Y":dbl, "X or R"=→"X":dbl, "waveform (Y)"=w407:waveform(dbl)[])  [unwired: 6 in, 1 out]
        n162 = Subtract(x=w414, y=w413) -> (x-y=w406:u64)
        n163 = call "fun_Adjust waveform t0.vi"("error in (no error)"=w411, "delta Timestamp(ticks)"=w406, "waveform (Y)"=w407, "Handle In"=w410) -> ("error out"=w408:errorcluster, "Adjusted Waveform"=w404:waveform(dbl)[], "Handle Out"=w409:T2)  [unwired: 5 in]
        n164 = case shown="0, Default" w405 {
          tunnel: w404 -> [w429 w430]
          frame 0, Default {
            "Plotter(XY)" <- w429
          }
          frame 1 {
            "Plotter(R&theta)" <- w430
          }
        }
        n165 = Bundle By Name(cluster=w415, "ZI Handle"=w409) -> (w417:T1)
        n166 = call <vilib>:"Clear Errors.vi"("error in (no error)"=w408) -> ("error out"=w426:errorcluster)  [unwired: 5 in, 1 out]
      }
      frame "FUN-Numeric_Stop" {
        n167 = Release Queue(queue=w432, error in (no error)=w433) -> (error out=w434:errorcluster)  [unwired: 1 in, 2 out]
      }
    }
  }
